vi "HEWH Create Multi Header.vi"(8 "error in (no error)":errorcluster, 11 "Array in":string[][](array[string])) -> (0 "error out":errorcluster, 3 "Array out":string[][](array[string]))   [LabVIEW 2019]
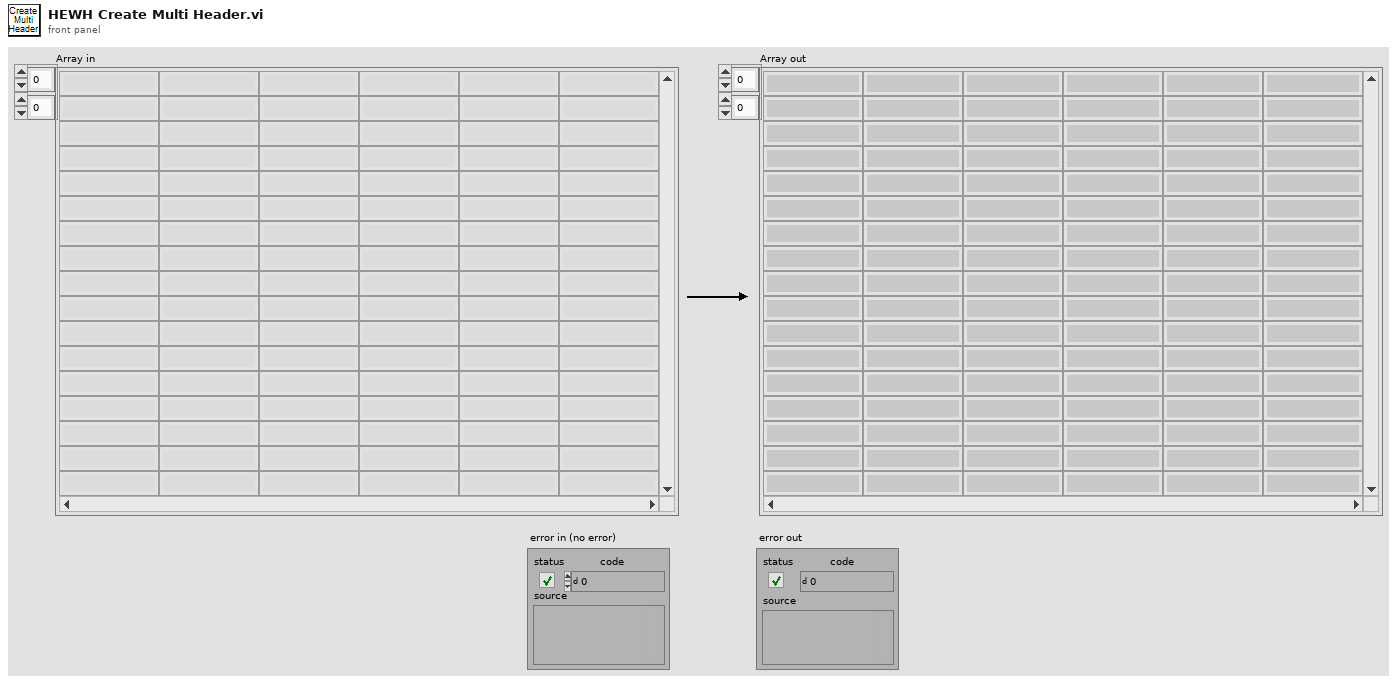
[diagram p1: front panel]
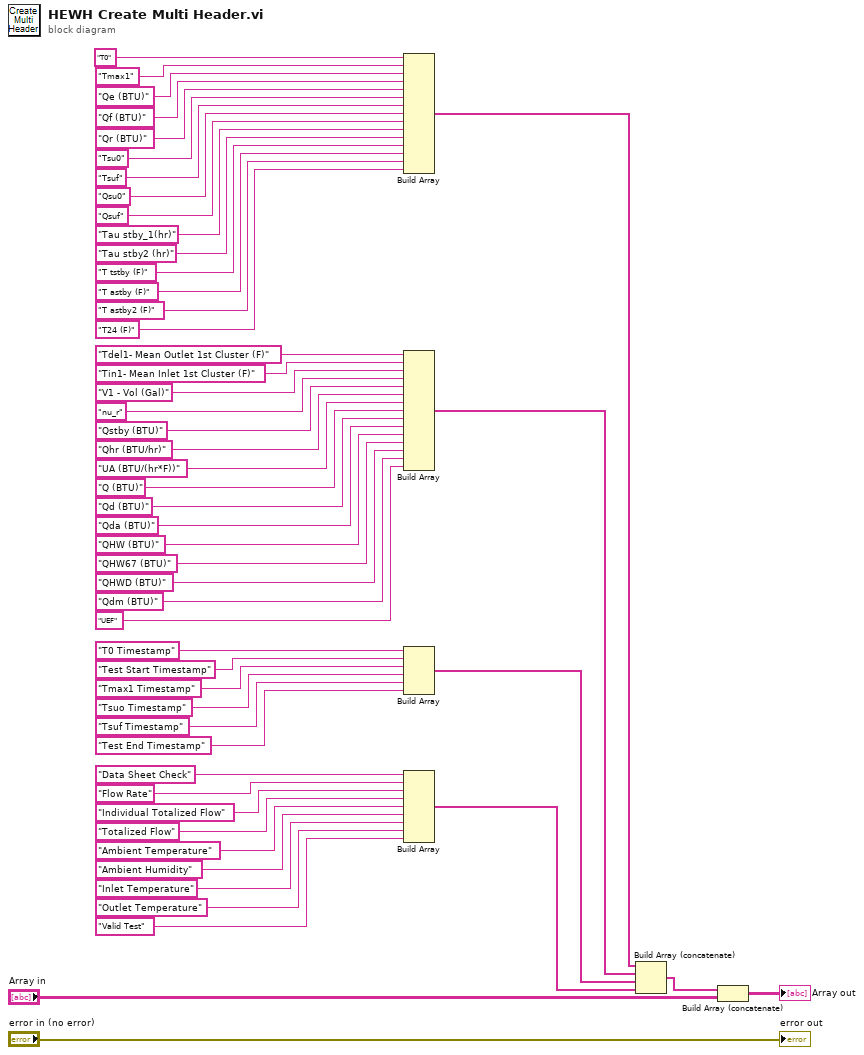
[diagram p0: block diagram]
diagram:
  n1 = Build Array("T0", "Tmax1", "Qe (BTU)", "Qf (BTU)", "Qr (BTU)", "Tsu0", "Tsuf", "Qsu0", "Qsuf", "Tau stby_1(hr)", "Tau stby2 (hr)", "T tstby (F)", "T astby (F)", "T astby2 (F)", "T24 (F)") -> (w50:string[])
  n2 = Build Array("Tdel1- Mean Outlet 1st Cluster (F)", "Tin1- Mean Inlet 1st Cluster (F)", "V1 - Vol (Gal)", "nu_r", "Qstby (BTU)", "Qhr (BTU/hr)", "UA (BTU/(hr*F))", "Q (BTU)", "Qd (BTU)", "Qda (BTU)", "QHW (BTU)", "QHW67 (BTU)", "QHWD (BTU)", "Qdm (BTU)", "UEF") -> (w51:string[])
  n3 = Build Array("T0 Timestamp", "Test Start Timestamp", "Tmax1 Timestamp", "Tsuo Timestamp", "Tsuf Timestamp", "Test End Timestamp") -> (w52:string[])
  n4 = Build Array("Data Sheet Check", "Flow Rate", "Individual Totalized Flow", "Totalized Flow", "Ambient Temperature", "Ambient Humidity", "Inlet Temperature", "Outlet Temperature", "Valid Test") -> (w53:string[])
  n5 = Build Array (concatenate)(w50, w51, w52, w53) -> (w3:string[])
  n6 = Build Array (concatenate)(w3, "Array in") -> (→"Array out":string[][])
  "error out" <- "error in (no error)"
